vi "Open Search Results Dialog.vi"(7 "VI Refnum":refnum<vi>, 8 "error in (no error)":errorcluster, 9 "Callers":T1, 10 "State":string, 11 "JKI SM in":refnum<class "JKI SM.lvclass">) -> (0 "error out":errorcluster)   [LabVIEW 2013]
uses:
  JKI State Machine API/source/Support/State Calls Array.ctl
  JKI State Machine API/source/Support/State Call Cluster.ctl
  JKI State Machine API/source/JKI SM/JKI SM.lvclass
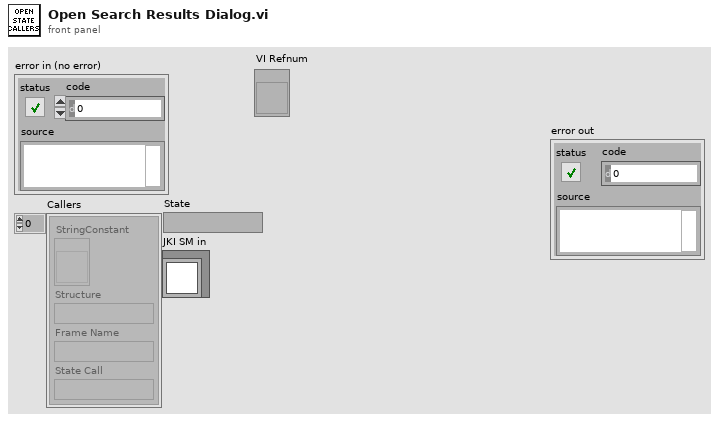
[diagram p1: front panel]
types:
  T1 = typedef "State Calls Array.ctl" = T2[]
  T2 = typedef "State Call Cluster.ctl" = cluster{"StringConstant":refnum<vi>, "Structure":string, "Frame Name":string, "State Call":string}
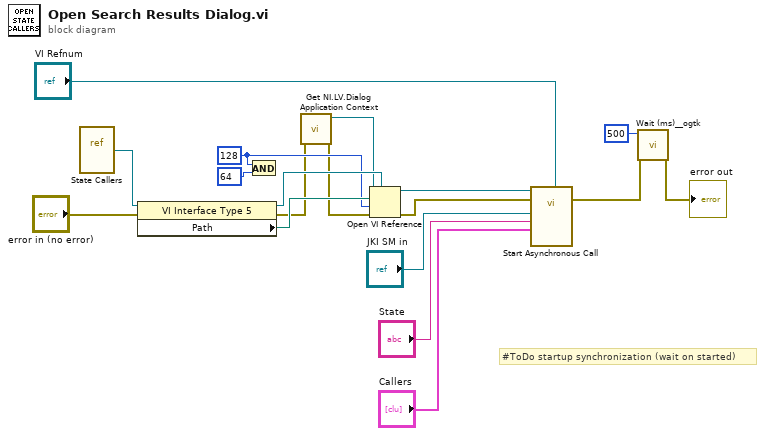
[diagram p0: block diagram]
diagram:
  w8 = 128 ("options")
  # "#ToDo startup synchronization (wait on started)"
  n1 = vi-ref "State Callers.vi"() -> (w18:refnum<vi>)
  n2 = property class="VI Interface Type 5"(reference=w18, error in="error in (no error)") -> (reference out=w14:refnum<vi>, error out=w3:errorcluster, "Path"=w17:path)
  n3 = And(x=w8, y=64 ("options")) -> ()  [unwired: 1 out]
  n4 = call "Get NI.LV.Dialog Application Context.vi"("error in (no error)"=w3) -> ("error out"=w2:errorcluster, "Application out"=w1:refnum<vi>)  [unwired: 9 in]
  n5 = Open VI Reference(type specifier VI Refnum (for type only)=w14, application reference (local)=w1, vi path=w17, options=w8, error in (no error)=w2) -> (vi reference=w15:refnum<vi>, error out=w9:errorcluster)  [unwired: 1 out]
  n6 = call-by-ref "Start Asynchronous Call"(reference=w15, error in=w9, "Calling VI Ref"="VI Refnum", "Callers"="Callers", "State"="State", "JKI SM in"="JKI SM in") -> (error out=w5:errorcluster)  [unwired: 7 in, 2 out]
  n7 = call <userlib>:"Wait (ms)__ogtk.vi"("error in (no error)"=w5, "milliseconds to wait"=u32 500) -> ("error out"=→"error out":errorcluster)  [unwired: 8 in, 1 out]
